vi "Get FPGA uService ID.vi"(8 "error in (no error)":errorcluster, 11 "Monkey in":refnum<class "Monkey.lvclass">) -> (0 "error out":errorcluster, 2 "FPGA uService ID":string, 3 "Monkey out":refnum<class "Monkey.lvclass">)   [LabVIEW 2020, in "Monkey.lvlib" / "Monkey.lvclass"]
uses:
  Monkey.lvclass
  Run Utilities/Run Instance/Run Instance.lvclass
  Support VIs/Global Memory.vi
  Run Utilities/Run Block/Run Block.lvclass
  Interfaces/FPGA Interface/FPGA Interface.lvclass
  TALOS.lvlib
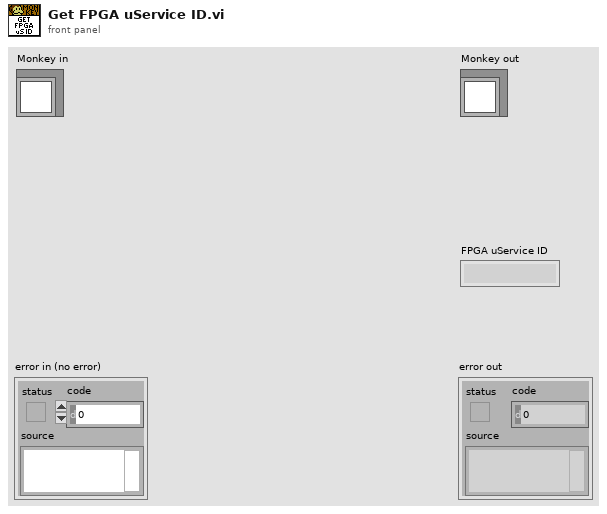
[diagram p1: front panel]
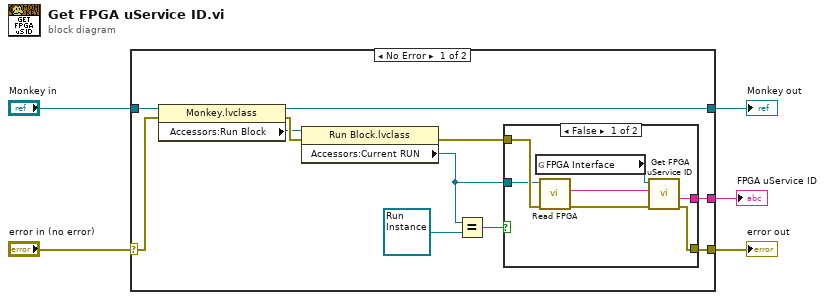
[diagram p0: block diagram]
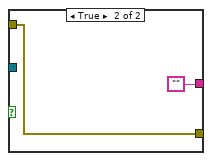
[diagram p2: hidden frame]
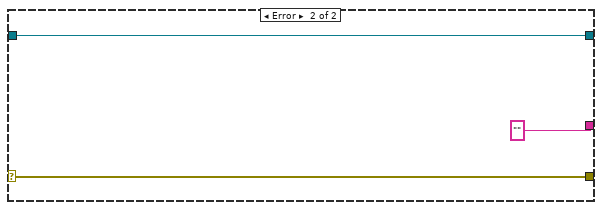
[diagram p3: hidden frame]
diagram:
  n1 = case shown="No Error" "error in (no error)" {
    selector: "error in (no error)" -> [w11 w28]
    tunnel: [w9 w28] -> w4
    tunnel: [w13 w27] -> w2
    tunnel: "Monkey in" -> [w14 w27]
    tunnel: [w10 "" ("uService ID")] -> w1
    frame No Error {
      n2 = property class="Monkey.lvclass"(reference=w14, error in=w11) -> (reference out=w13:refnum<class "Monkey.lvclass">, error out=w15:errorcluster, "Accessors:Run Block"=w12:refnum<class "Run Block.lvclass">)
      n3 = property class="Run Block.lvclass"(reference=w12, error in=w15) -> (error out=w16:errorcluster, "Accessors:Current RUN"=w8:refnum<class "Run Instance.lvclass">)  [unwired: 1 out]
      n4 = Equal?(x=w8, y=refnum<class "Run Instance.lvclass"> refnum) -> (x = y?=w6:bool)
      n5 = case shown="False" w6 {
        tunnel: w16 -> [w23 w25]
        tunnel: [w22 ""] -> w10
        tunnel: [w21 w25] -> w9
        tunnel: w8 -> [w17 _]
        frame False {
          n6 = global read "Global Memory.vi" "FPGA Interface"() -> (w20:refnum<class "FPGA Interface.lvclass">)
          n7 = call-dynamic "Read FPGA.vi"("error in (no error)"=w23, "Run Instance in"=w17) -> ("error out"=w18:errorcluster, "FPGA Name"=w19:string)  [unwired: 7 in, 1 out]
          n8 = call-dynamic "Get FPGA uService ID.vi"("error in"=w18, "FPGA Name"=w19, "FPGA Interface"=w20) -> ("error out"=w21:errorcluster, "uService ID"=w22:string)  [unwired: 4 in, 1 out]
        }
        frame True {
        }
      }
    }
    frame Error {
    }
  }
  "error out" <- w4
  "Monkey out" <- w2
  "FPGA uService ID" <- w1
